vi "Pin Width_Pixel Intensity Determination.vi"(8 "error in":errorcluster, 10 "Image":T1, 11 "Column Number from Edge Detection":i32) -> (0 "error out":errorcluster, 3 "Number of Dark Pixels from the edge":dbl)   [LabVIEW 2016]
uses:
  <vilib>/vision/Image Controls.llb/IMAQ Image.ctl
  <vilib>/vision/NI_Vision_Development_Module.lvlib
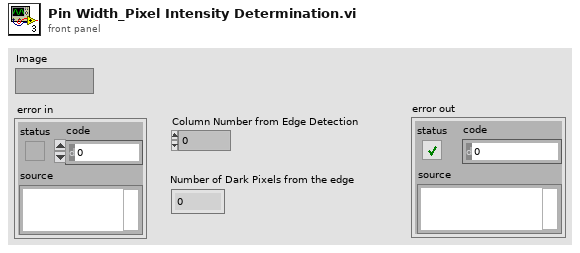
[diagram p1: front panel]
types:
  T1 = typedef "IMAQ Image.ctl" = refnum<image>
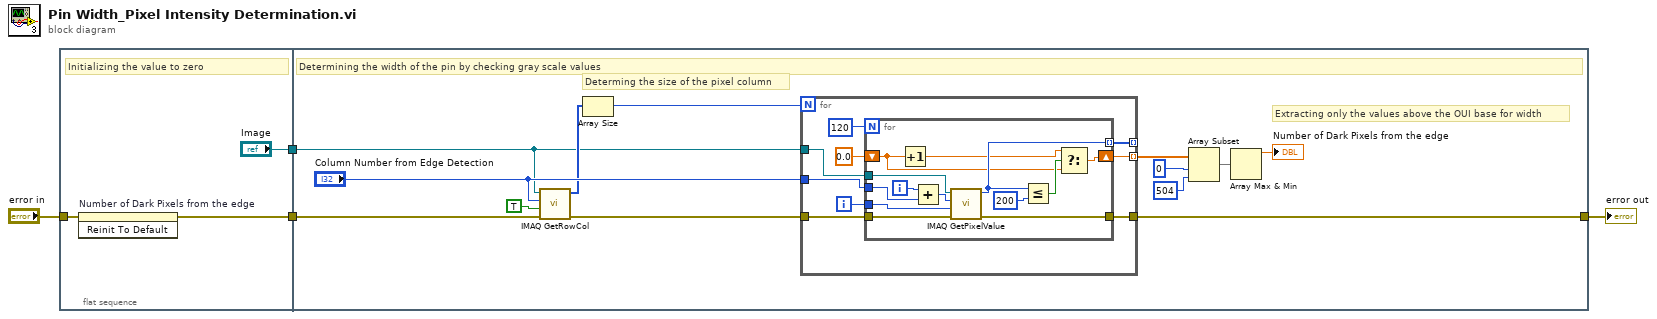
[diagram p0: block diagram]
diagram:
  n1 = flat-sequence {
    tunnel: "error in" -> [w7]
    tunnel: [w6] -> w3
    tunnel: ["Image"] -> w2
    tunnel: w3 -> [w10]
    tunnel: w2 -> [w8]
    tunnel: [w9] -> w1
    frame #0 {
      # "Initializing the value to zero"
      n2 = invoke on="Number of Dark Pixels from the edge" class="DigNum (strict)" method="Reinit To Default"(error in=w7) -> (error out=w6:errorcluster)  [unwired: 2 in, 2 out]
    }
    frame #1 {
      # "Extracting only the values above the OUI base for width"
      # "Determing the size of the pixel column"
      # "Determining the width of the pin by checking gray scale values"
      n3 = call "IMAQ GetRowCol"("Image"=w8, "Number"="Column Number from Edge Detection", "Row / Column (Row)"=TRUE, "error in (no error)"=w10) -> ("Pixels (U8)"=w12:u8[], "error out"=w14:errorcluster)  [unwired: 2 in, 3 out]
      n4 = Array Size(array=w12) -> (size(s)=w13:i32)
      n5 = for {
        N: w13 -> [_]
        tunnel: w14 -> [w28]
        tunnel: [w27] -> w9
        tunnel: [w26] -> _ mode=indexing
        tunnel: [w23] -> w17 mode=indexing
        tunnel: "Column Number from Edge Detection" -> [w22]
        tunnel: w8 -> [w21]
        i -> [w29]
        n6 = for {
          N: 120 -> [_]
          tunnel: w29 -> [w42]
          tunnel: w28 -> [w41]
          tunnel: [w40] -> w27
          tunnel: [w39] -> w26 mode=indexing
          shift-right: [w35] -> w23
          shift-left: 0.0 -> [w34]
          tunnel: w22 -> [w32]
          tunnel: w21 -> [w30]
          i -> [w33]
          n7 = Increment(x=w34) -> (x+1=w36:dbl)
          n8 = Add(x=w33, y=w32) -> (x+y=w31:i32)
          n9 = call "IMAQ GetPixelValue"("Image"=w30, "X Coordinate"=w31, "Y Coordinate"=w42, "error in (no error)"=w41) -> ("Pixel Value (U8)"=w39:u8, "error out"=w40:errorcluster)  [unwired: 2 in, 3 out]
          n10 = Less Or Equal?(x=w39, y=u8 200) -> (x <= y?=w38:bool)
          n11 = Select(t=w36, s=w38, f=w34) -> (s? t:f=w35:dbl)
        }
      }
      n12 = Array Subset(array=w17, index=0, length=504) -> (w18:dbl[])
      n13 = Array Max & Min(array=w18) -> (max value=→"Number of Dark Pixels from the edge":dbl)  [unwired: 3 out]
    }
  }
  "error out" <- w1
